vi "Quotient Remainder solution.vi"() -> ()   [LabVIEW 2018]
uses:
  ctl/Coin data--cluster.ctl
panel:
  out "No. Solutions":i32
  out "Goal amount (p)":i32=1199
  out "Quantities":i32[](array[numeric])
  out "Quantities that yield goal":i32[][](array[numeric])
  out "Values (p)":i32[](array[numeric])
  # "Beer money - Quotient Remainder Solution"
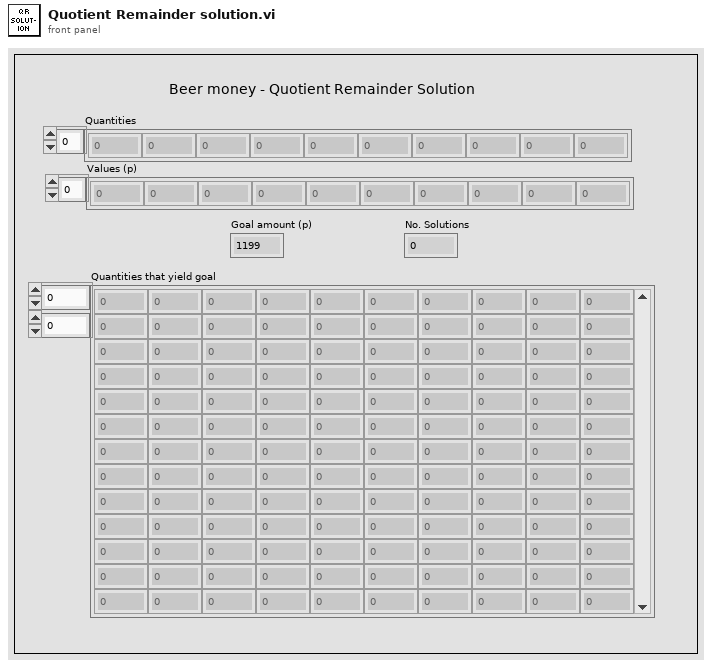
[diagram p1: front panel]
types:
  T1 = typedef "Coin data--cluster.ctl" = cluster{"Coin/note":i32, "Quantity":i32}
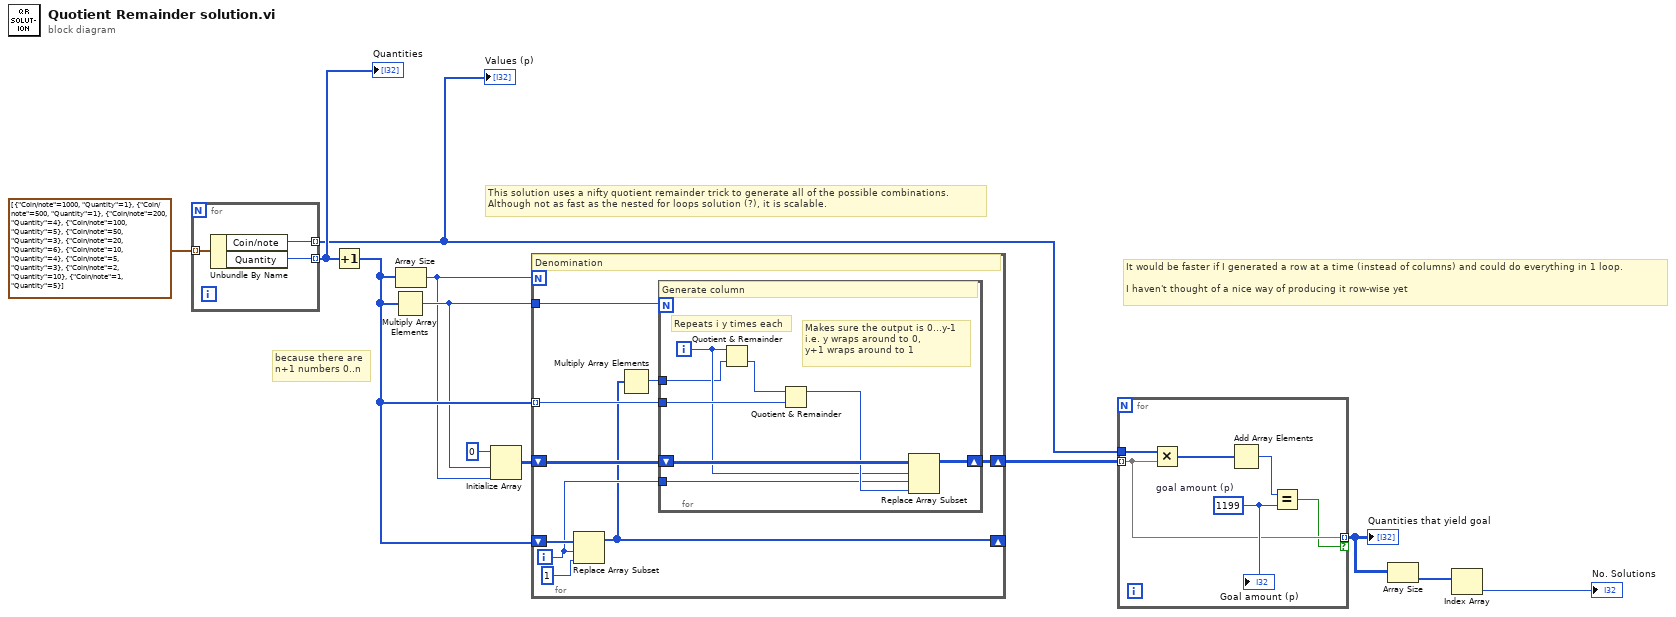
[diagram p0: block diagram]
diagram:
  # "This solution uses a nifty quotient remainder trick to generate all of the possible combinations.\nAlthough not as fast as the nested for loops solution (?), it is scalable."
  # "It would be faster if I generated a row at a time (instead of columns) and could do everything in 1 loop.\n\nI haven't thought of a nice way of producing it row-wise yet"
  # "because there are \nn+1 numbers 0..n"
  n1 = for {
    tunnel: [w15] -> w5 mode=indexing
    tunnel: [w14] -> w12 mode=indexing
    tunnel: T1[] [{"Coin/note"=1000, "Quantity"=1}, {"Coin/note"=500, "Quantity"=1}, {"Coin/note"=200, "Quantity"=4}, {"Coin/note"=100, "Quantity"=5}, {"Coin/note"=50, "Quantity"=3}, {"Coin/note"=20, "Quantity"=6}, {"Coin/note"=10, "Quantity"=4}, {"Coin/note"=5, "Quantity"=3}, {"Coin/note"=2, "Quantity"=10}, {"Coin/note"=1, "Quantity"=5}] -> [w13] mode=indexing
    n2 = Unbundle By Name(w13) -> ("Coin/note"=w15:i32, "Quantity"=w14:i32)
  }
  "Values (p)" <- w5
  "Quantities" <- w12
  n3 = Increment(x=w12) -> (x+1=w11:i32[])
  n4 = Multiply Array Elements(1:w11) -> (0:w9:i32)
  n5 = Array Size(array=w11) -> (size(s)=w8:i32)
  n6 = Initialize Array(0 ("product"), w9, w8) -> (w7:i32[][])
  n7 = for {
    N: w8 -> [_]
    tunnel: w9 -> [w24]
    tunnel: w11 -> [w23] mode=indexing
    shift-right: [w16] -> _
    shift-left: w11 -> [w20]
    shift-right: [w21] -> w6
    shift-left: w7 -> [w22]
    i -> [w18]
    # "Denomination"
    n8 = Replace Array Subset(array=w20, new element=1 ("new element/subarray"), index=w18) -> (w16:i32[])
    n9 = Multiply Array Elements(1:w16) -> (0:w17:i32)
    n10 = for {
      N: w24 -> [_]
      tunnel: w23 -> [w31]
      shift-right: [w29] -> w21
      shift-left: w22 -> [w30]
      tunnel: w18 -> [w26]
      tunnel: w17 -> [w25]
      i -> [w27]
      # "Makes sure the output is 0...y-1\ni.e. y wraps around to 0,\ny+1 wraps around to 1"
      # "Repeats i y times each"
      # "Generate column"
      n11 = Quotient & Remainder(x=w27, y=w25) -> (floor(x/y)=w32:i32)  [unwired: 1 out]
      n12 = Quotient & Remainder(x=w32, y=w31) -> (x-y*floor(x/y)=w28:i32)  [unwired: 1 out]
      n13 = Replace Array Subset(array=w30, new element=w28, index (row)=w27, index (col)=w26) -> (w29:i32[][])
    }
  }
  n14 = for {
    tunnel: w6 -> [w34] mode=indexing
    tunnel: w5 -> [w35]
    tunnel: [w34] -> w4 mode=indexing if=w33
    w36 = 1199  # goal amount (p)
    n15 = Multiply(x=w35, y=w34) -> (x*y=w37:i32[])
    n16 = Add Array Elements(numeric array=w37) -> (sum=w38:i32)
    n17 = Equal?(x=w38, y=w36) -> (x = y?=w33:bool)
    "Goal amount (p)" <- w36
  }
  "Quantities that yield goal" <- w4
  n18 = Array Size(array=w4) -> (size(s)=w3:i32[])
  n19 = Index Array(array=w3) -> (element=→"No. Solutions":i32)  [unwired: 1 in]
